vi "lia_fpga2.vi"() -> ()   [LabVIEW 2009]
uses:
  <vilib>/Platform/TimedLoop/XDataNode/XDataNode.xnode
  <vilib>/Platform/TimedLoop/XDataNode/loadlvalarms.vi
  <vilib>/Platform/TimedLoop/XDataNode/timing_clust.ctl
  <vilib>/Platform/TimedLoop/XDataNode/nitl_modes.ctl
  <vilib>/Platform/TimedLoop/XDataNode/wakeup.ctl
  <vilib>/rvi/DataTransferAndStorage/Container/XNode/niFpgaContainer.xnode
  <vilib>/rvi/FIFO/Fifo_Resource/nirvififoUniquifyingName.vi
  <vilib>/eio/EIONode/EIONode.xnode
  <vilib>/rvi/eio/nirviEIOImplementation/nirviEIOImplementation.xnode
  <vilib>/rvi/eio/common/nirviEmuTemplateMethod_noerrors.vi
  <vilib>/rvi/eio/common/nirviEmuClasses.ctl
  <vilib>/rvi/LocalResourceManager/LocalResourceManager.xnode
  <vilib>/rvi/eio/common/nirviEmuReportErrorAndStop.vi
  <vilib>/rvi/DataTransferAndStorage/Container/Common/niFpgaContainerSetEmuInfo.vi
  <vilib>/rvi/DataTransferAndStorage/Container/Common/niFpgaContainerState.ctl
  <vilib>/rvi/DataTransferAndStorage/Container/Common/niFpgaDataTypeControl.ctl
  <vilib>/rvi/DataTransferAndStorage/Container/Common/niFpgaContainerImplementationControl.ctl
  <vilib>/rvi/DataTransferAndStorage/Container/Common/niFpgaContainerArbitrationOptionsControl.ctl
  <vilib>/rvi/DataTransferAndStorage/Container/Common/niFpgaTransferTypeControl.ctl
  <vilib>/rvi/DataTransferAndStorage/Container/Common/niFpgaContainerInitializationParameters.ctl
  <vilib>/rvi/DataTransferAndStorage/Container/Common/niFpgaContainerMetaDataKey.ctl
  <vilib>/Platform/TimedLoop/XDataNode/XDNodeRunTimeDep.lvlib
panel:
  in  "beta":i16
  in  "stop 2":bool
  out "fifo":i16
  in  "stop":bool
  in  "stages":i32
  in  "dec":i32
  in  "dec2":i32
  in  "dec1":i32
  in  "decimation":i32
  out "Actual Gen Rate (ticks)":u32
  in  "Update Rate (ticks)":u32
  out "Accumulator Value":u32
  in  "Signal Amplitude":u16
  in  "Phase Shift":u32
  in  "Accumulator Increment":u32
  in  "Reset Accumulator":bool
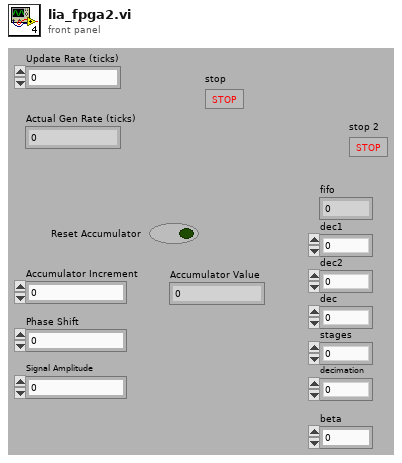
[diagram p1: front panel]
types:
  T1 = typedef "nirviEmuClasses.ctl" = enum16{"IO Read", "IO Write", "Method", "Property Read", "Property Write"}
  T2 = typedef "XDNodeRunTimeDep.lvlib/timing_clust.ctl" = cluster{"Expected End [f-1]":u64, "Actual End [f-1]":u64, "Finished Late? [f-1]":bool, "Expected End [i-1]":u64, "Actual End [i-1]":u64, "Finished Late? [i-1]":bool, "Expected Start [i]":u64, "Actual Start [i]":u64, "Expected Start [f]":u64, "Actual Start [f]":u64, "Source Name":string, "Structure Name":string, "Period":i64, "Deadline":i64, "Offset":i64, "Start":i64, "Priority":i32, "Timeout":i32, "Mode":T3, "Wakeup Reason":T4, "Error":errorcluster, "Source Type":string, "Secondary Source Type":string, "Global End Time":u64, "Global Start Time":u64, "Frame Duration":u64, "Iteration Duration":u64, "Assigned CPU":i32, "I/O Scan Engine Mode":u32}
  T3 = typedef "XDNodeRunTimeDep.lvlib/nitl_modes.ctl" = enum32{"No Change", "Process missed periods, maintain original phase", "Discard missed periods, maintain original phase", "Process missed periods, ignore original phase", "Discard missed periods, ignore original phase"}
  T4 = typedef "XDNodeRunTimeDep.lvlib/wakeup.ctl" = enum32{"Normal", "Aborted", "Asynchronous wakeup", "Timing source error", "Timed loop error", "Timeout"}
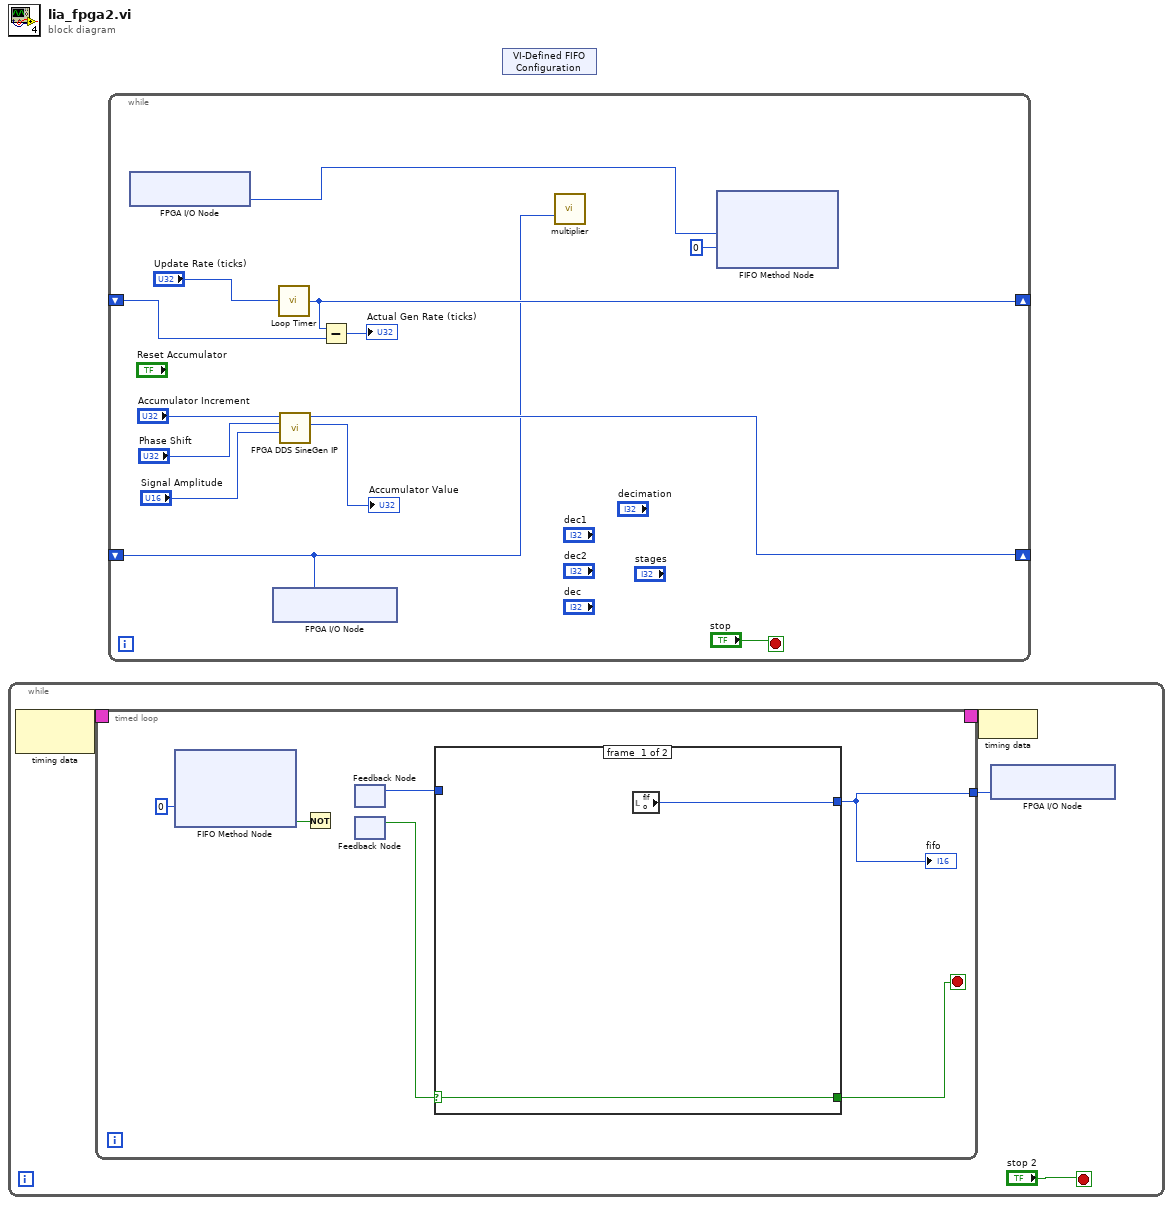
[diagram p0: block diagram]
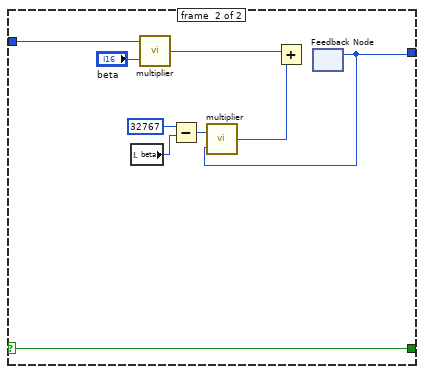
[diagram p2: hidden frame]
diagram:
  n1 = while {
    stop <- "stop 2" stop-if-true
    n2 = node-c288() -> (w4:T2)  [unwired: 1 in]
    n3 = timed-loop {
      timing: w4 -> [_]
      timing-out: [_] -> w3
      tunnel: [w18] -> w1
      stop <- w19 stop-if-true
      n4 = xnode ("FIFO Method Node")("Timeout"=0) -> ("Element"=w17:i16, "Timed Out?"=w22:bool)  [unwired: 1 in, 1 out]
      n5 = Not(x=w22) -> (.not. x?=w21:bool)
      n6 = feedback #1() -> (w16:i16)  [unwired: 1 in]
      n7 = feedback #2() -> (w20:bool)  [unwired: 1 in]
      n8 = case shown="True" w20 {
        selector: w20 -> [w24 w35]
        tunnel: [w25 w26] -> w18
        tunnel: [w24 w35] -> w19
        tunnel: w16 -> [_ w34]
        frame #0 {
          n9 = local read "fifo"() -> (w25:i16)
        }
        frame #1 {
          n10 = local read "beta"() -> (w30:i16)
          n11 = call "multiplier.vi"("Y"="beta", "X"=w34) -> ("XY"=w32:i16)
          n12 = Subtract(x=i16 32767, y=w30) -> (x-y=w27:i16)
          n13 = feedback #3() -> (w26:i16)  [unwired: 1 in]
          n14 = call "multiplier.vi"("Y"=w26, "X"=w27) -> ("XY"=w29:i16)
          n15 = Add(x=w32, y=w29) -> (x+y=w28:i16)
        }
      }
      "fifo" <- w18
    }
    n16 = node-c288(w3) -> ()
    n17 = xnode "FPGA I/O Node"("Connector0/AO1"=w1) -> ()  [unwired: 1 in, 1 out]
  }
  n18 = while {
    shift-right: [w96] -> _
    shift-left: _ -> [w90]
    shift-right: [w94] -> _
    shift-left: _ -> [w92]
    stop <- "stop" stop-if-true
    n19 = xnode "FPGA I/O Node"() -> ("Connector0/AI0"=w88:i16)  [unwired: 1 in, 1 out]
    n20 = xnode "FPGA I/O Node"("Connector0/AO0"=w90) -> ()  [unwired: 1 in, 1 out]
    n21 = call "Loop Timer"("Count(Ticks)"="Update Rate (ticks)") -> ("Tick Count(Ticks)"=w94:u32)
    n22 = call "FPGA DDS SineGen IP.vi"("Signal Amplitude (x 2^15)"="Signal Amplitude", "Phase Shift"="Phase Shift", "Accumulator Increment"="Accumulator Increment") -> ("Accumulator Value"=→"Accumulator Value":u32, "Signal Value"=w96:i16)  [unwired: 7 in]
    n23 = Subtract(x=w94, y=w92) -> (x-y=→"Actual Gen Rate (ticks)":u32)
    n24 = call "multiplier.vi"("Y"=w90) -> ()  [unwired: 1 in, 1 out]
    n25 = xnode ("FIFO Method Node")("Element"=w88, "Timeout"=0) -> ()  [unwired: 1 in, 2 out]
  }
  n26 = xnode "VI-Defined FIFO Configuration"() -> ()  [unwired: 1 out]
